vi "Get_data_for_OE.vi"(7 "Station no.":i32, 8 "error in (no error)":errorcluster, 9 "Shift":string, 10 "Date":timestamp, 11 "Refnum in":T1) -> (0 "error out":errorcluster, 1 "Rejected Product Data":string[][](array[string]), 2 "data":string[][](array[string]), 3 "resulting string":string)   [LabVIEW 2017]
uses:
  <vilib>/addons/database/Connection.llb/Conn ObjectReference.ctl
  <vilib>/addons/database/_DB Variant To Data/Database Variant To Data.xnode
  <vilib>/addons/database/NI_Database_API.lvlib
panel:
  out "Sorted Pointers 2":i32[](array[numeric])
  in  "Order":enum16{"ascending", "descending"}(ring)
  out "sorted array 2":timestamp[](array[timestamp])
  in  "Array":timestamp[](array[timestamp])
  out "resulting string 2":string
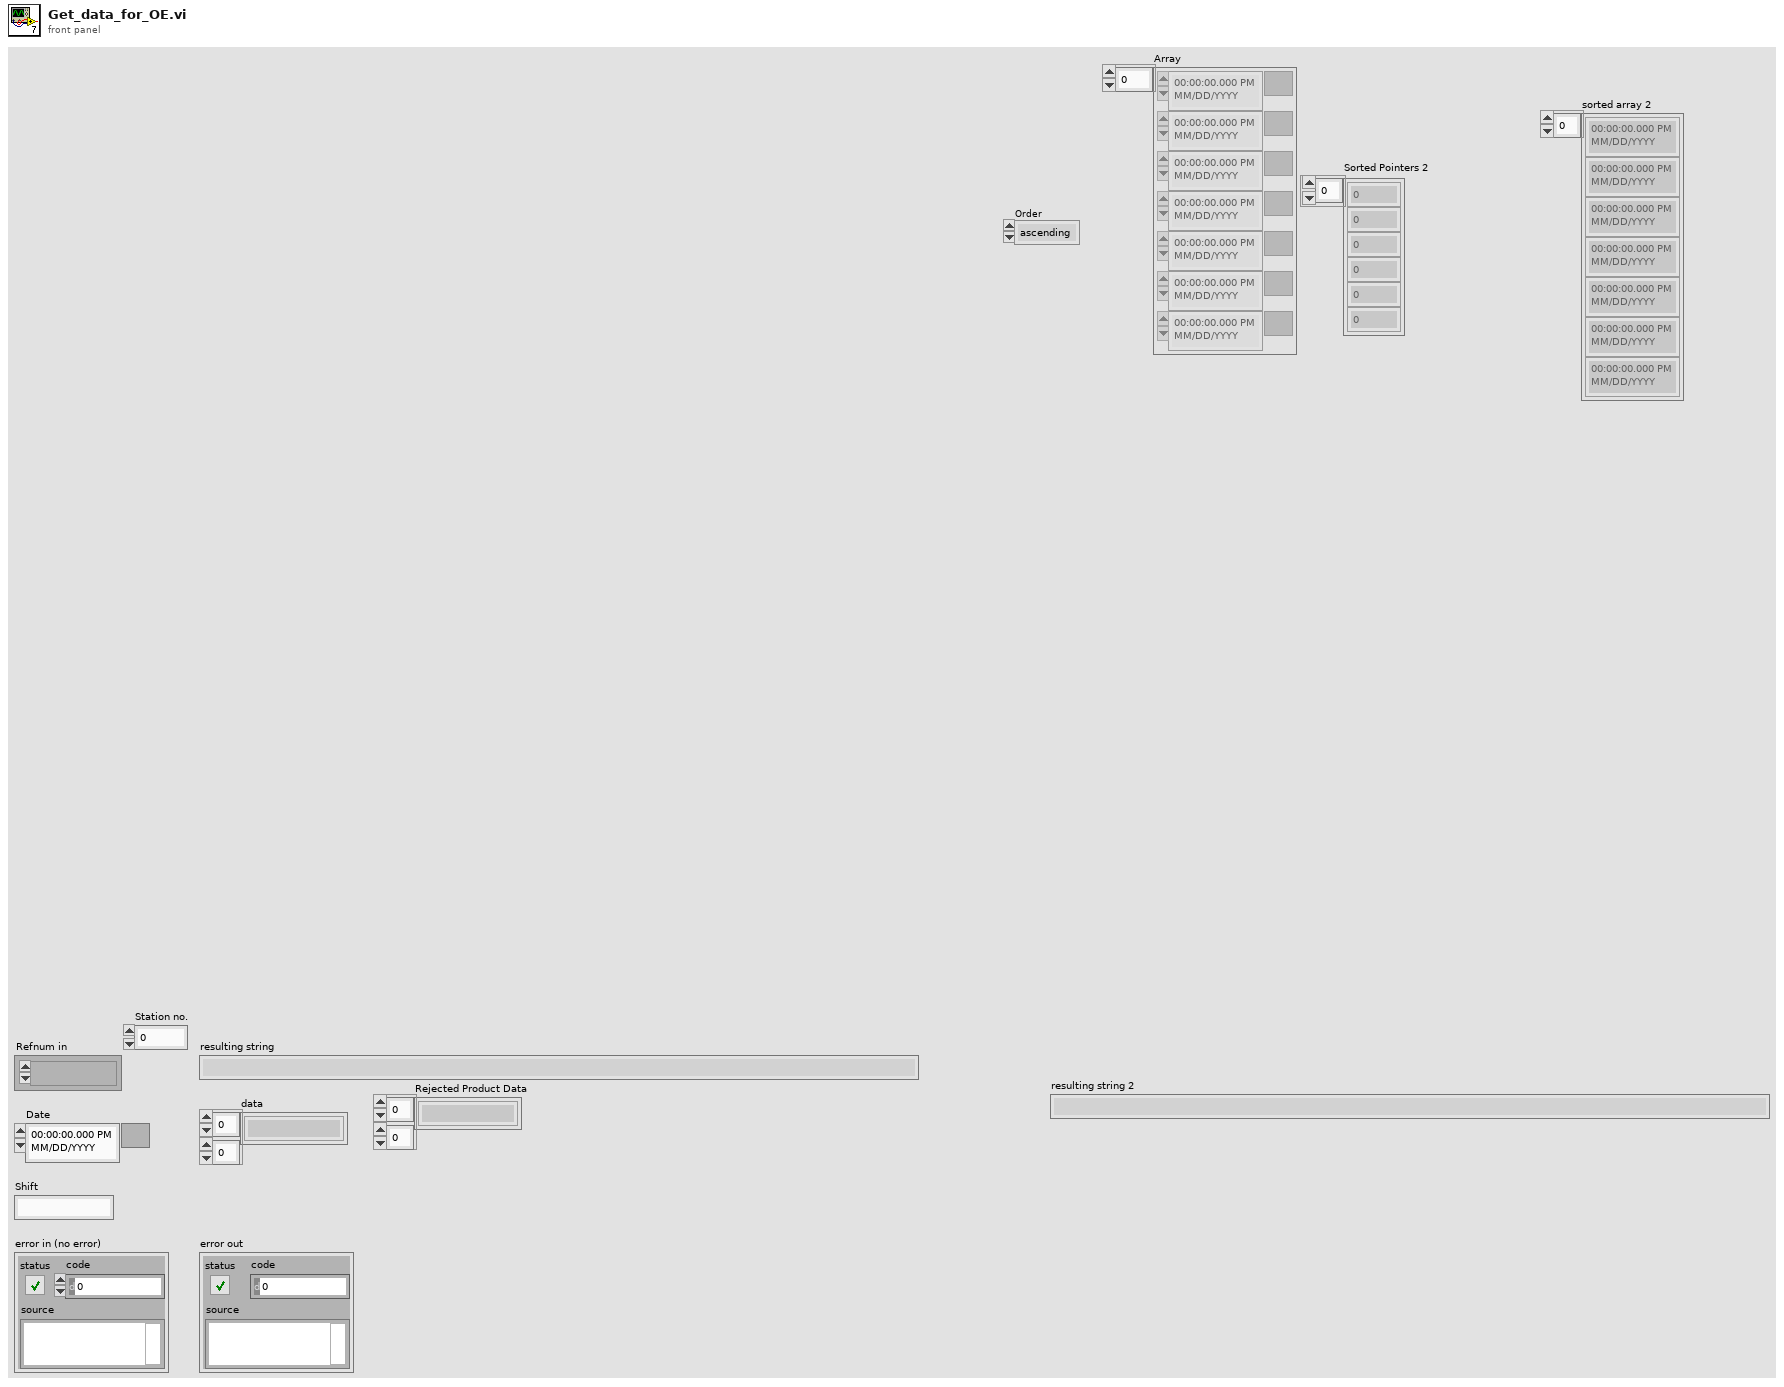
[diagram p1: front panel]
types:
  T1 = typedef "NI_Database_API.lvlib/Conn ObjectReference.ctl" = refnum<k1>
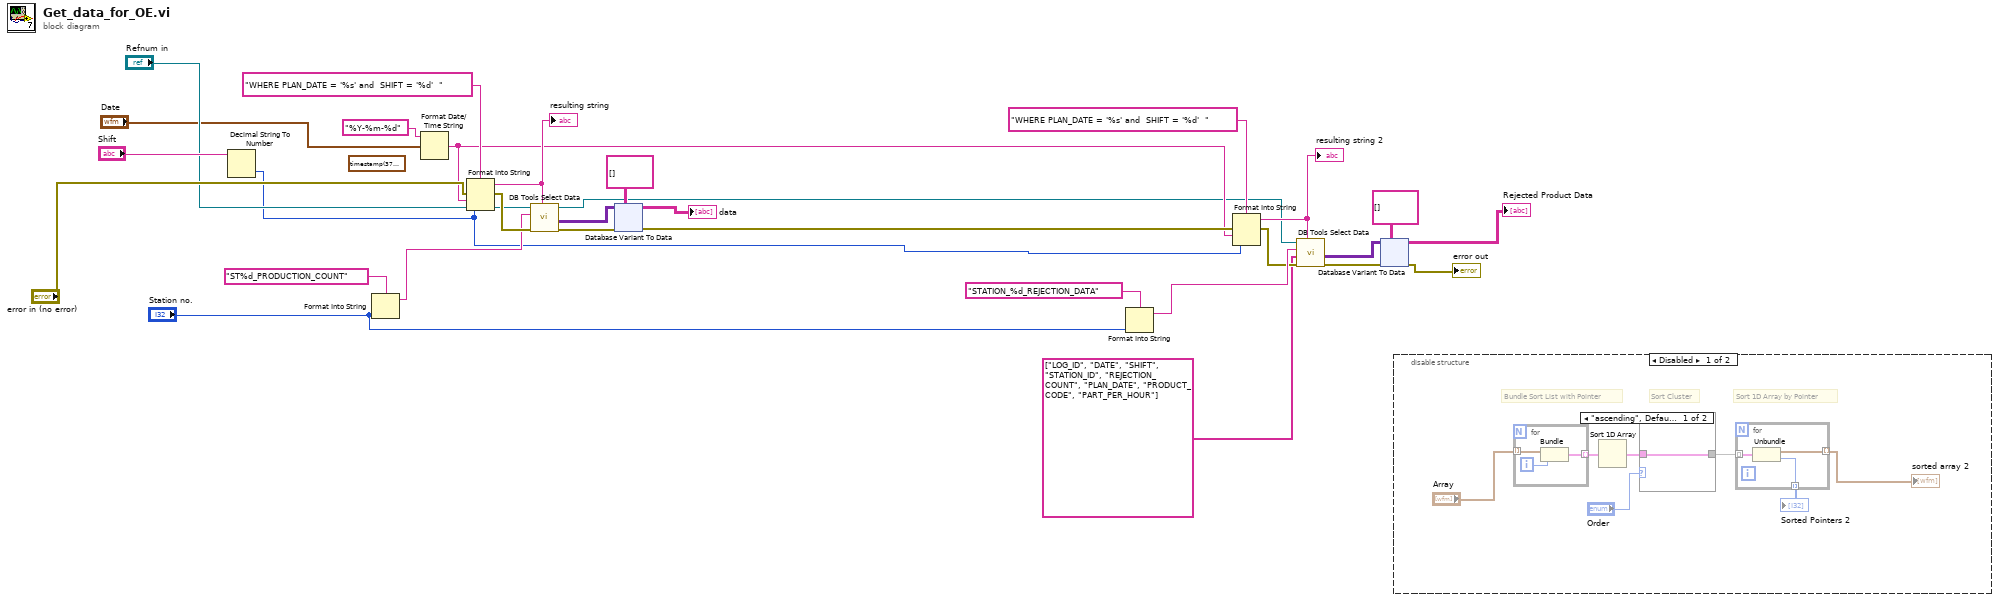
[diagram p0: block diagram]
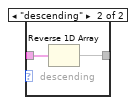
[diagram p2: hidden frame]
diagram:
  (unwired) timestamp(3772310400 s since 1904-01-01) ("Date")
  n1 = Decimal String To Number(string="Shift") -> (number=w5:i32)  [unwired: 2 in, 1 out]
  n2 = Format Into String(format string="ST%d_PRODUCTION_COUNT" ("table"), "Station no.") -> (resulting string=w18:string)  [unwired: 2 in, 1 out]
  n3 = Format Date/Time String(time format string (%c)="%Y-%m-%d", seconds (now)="Date") -> (date/time string=w3:string)  [unwired: 1 in]
  n4 = Format Into String(format string="WHERE PLAN_DATE = '%s' and  SHIFT = '%d'  ", error in="error in (no error)", w3, w5) -> (resulting string=w27:string, error out=w30:errorcluster)  [unwired: 1 in]
  "resulting string" <- w27
  n5 = call <vilib>:"DB Tools Select Data.vi"("condition"=w27, "error in (no error)"=w30, "table"=w18, "connection reference"="Refnum in") -> ("error out"=w21:errorcluster, "data"=w22:variant[][], "connection reference out"=w1:T1)  [unwired: 2 in]
  n6 = xnode "Database Variant To Data"("database variant"=w22, "error in (no error)"=w21, "type"=string[][] [] ("Elements Found")) -> ("data"=→"data":string[][], "error out"=w8:errorcluster)
  n7 = Format Into String(format string="STATION_%d_REJECTION_DATA" ("table"), "Station no.") -> (resulting string=w17:string)  [unwired: 2 in, 1 out]
  n8 = Format Into String(format string="WHERE PLAN_DATE = '%s' and  SHIFT = '%d'  ", error in=w8, w3, w5) -> (resulting string=w12:string, error out=w10:errorcluster)  [unwired: 1 in]
  "resulting string 2" <- w12
  n9 = call <vilib>:"DB Tools Select Data.vi"("condition"=w12, "error in (no error)"=w10, "columns"=string[] ["LOG_ID", "DATE", "SHIFT", "STATION_ID", "REJECTION_COUNT", "PLAN_DATE", "PRODUCT_CODE", "PART_PER_HOUR"] ("columns 3"), "table"=w17, "connection reference"=w1) -> ("error out"=w15:errorcluster, "data"=w14:variant[][])  [unwired: 1 in, 1 out]
  n10 = xnode "Database Variant To Data"("database variant"=w14, "error in (no error)"=w15, "type"=string[][] [] ("Elements Found")) -> ("data"=→"Rejected Product Data":string[][], "error out"=→"error out":errorcluster)
  n11 = disable-structure shown="Disabled" {
    frame Disabled {
      # "Sort 1D Array by Pointer"
      # "Sort Cluster"
      # "Bundle Sort List with Pointer"
      n12 = for {
        tunnel: "Array" -> [w40] mode=indexing
        tunnel: [w38] -> w35 mode=indexing
        i -> [w39]
        n13 = Bundle("Time Stamp"=w40, w39) -> (w38:cluster{"Time Stamp":timestamp, i32})  [unwired: 1 in]
      }
      n14 = Sort 1D Array(array=w35) -> (sorted array=w34:cluster{"Time Stamp":timestamp, i32}[])
      n15 = case shown="\"ascending\", Default" "Order" {
        tunnel: [w41 w42] -> w36
        tunnel: w34 -> [w41 w43]
        frame "ascending", Default {
        }
        frame "descending" {
          # "descending"
          n16 = Reverse 1D Array(array=w43) -> (reversed array=w42:cluster{"Time Stamp":timestamp, i32}[])
        }
      }
      n17 = for {
        tunnel: w36 -> [w46] mode=indexing
        tunnel: [w44] -> w31 mode=indexing
        tunnel: [w45] -> w33 mode=indexing
        n18 = Unbundle(w46) -> ("Time Stamp"=w44:timestamp, w45:i32)
      }
      "sorted array 2" <- w31
      "Sorted Pointers 2" <- w33
    }
    frame Enabled {
    }
  }
